vi "testF710.vi"() -> ()   [LabVIEW 2019]
uses:
  <vilib>/Instr/_visa.llb/Select Event Type.ctl
panel:
  out "data buffer":u8[](array[numeric])
  in  "stop":bool
  out "Event Type":T1=1073684491 items=["Service Request"=1073684491, "Trigger"=3221168138, "Clear"=1073684493, "VXI Signal"=1073684512, "VXI/VME Interrupt"=3221168161, "VXI/VME Sysfail"=1073684509, "VXI/VME Sysreset"=1073684510, "GPIB CIC"=1073684498, "GPIB Talk"=1073684499, "GPIB Listen"=1073684500, "PXI Interrupt"=1073684514, "Serial Break"=1073684515, "Serial TermChar"=1073684516, "Serial CTS"=1073684521, "Serial DSR"=1073684522, "Serial DCD"=1073684524, "Serial RI"=1073684526, "Serial Character"=1073684533, "USB Interrupt"=1073684535, "All Enabled"=1073709055]
  out "error out":errorcluster
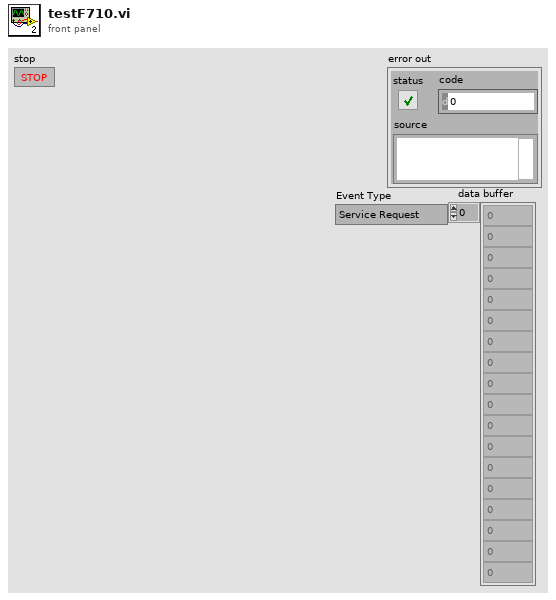
[diagram p1: front panel]
types:
  T1 = typedef "Select Event Type.ctl" = u32
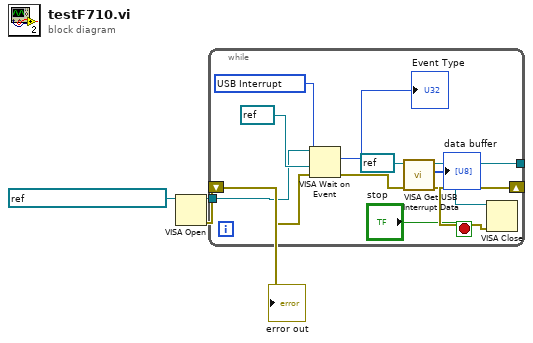
[diagram p0: block diagram]
diagram:
  n1 = VISA Open(VISA resource name=refnum<visa-resource-name> "USB0::0x046D::0xC21F::608C9160::RAW") -> (VISA resource name=w2:refnum<visa-resource-name>, error out=w1:errorcluster)  [unwired: 4 in]
  "error out" <- w1
  n2 = while {
    tunnel: [w11] -> w3
    tunnel: w2 -> [w9]
    shift-right: [w13] -> w4
    shift-left: w1 -> [w8]
    stop <- "stop" stop-if-true
    w15 = T1 1073684535 items=["Service Request"=1073684491, "Trigger"=3221168138, "Clear"=1073684493, "VXI Signal"=1073684512, "VXI/VME Interrupt"=3221168161, "VXI/VME Sysfail"=1073684509, "VXI/VME Sysreset"=1073684510, "GPIB CIC"=1073684498, "GPIB Talk"=1073684499, "GPIB Listen"=1073684500, "PXI Interrupt"=1073684514, "Serial Break"=1073684515, "Serial TermChar"=1073684516, "Serial CTS"=1073684521, "Serial DSR"=1073684522, "Serial DCD"=1073684524, "Serial RI"=1073684526, "Serial Character"=1073684533, "USB Interrupt"=1073684535, "All Enabled"=1073709055] ("Event Type")
    n3 = VISA Wait on Event(8:w8, 9:refnum<visa-resource-name> refnum ("event class (Generic Event)"), 10:w15, 11:w9) -> (0:w14:errorcluster, 2:→"Event Type":u32)  [unwired: 1 in, 2 out]
    n4 = call <vilib>:"VISA Get USB Interrupt Data.vi"("error in (no error)"=w14, "VISA USB Intr Event"=refnum<visa-resource-name> refnum) -> ("error out"=w13:errorcluster, "data buffer"=→"data buffer":u8[], "VISA USB Intr Event out"=w11:refnum<visa-resource-name>)  [unwired: 7 in]
  }
  n5 = VISA Close(VISA resource name=w3, error in (no error)=w4) -> ()  [unwired: 1 out]
